vi "Strafe Correction.vi"() -> ()   [LabVIEW 2018]
uses:
  Global Variables/Yaw.vi
  Global Variables/Strafe Correction TF.vi
  Global Variables/Follow Yaw.vi
  Global Variables/Strafe Correction Voltage.vi
  <vilib>/addons/control/pid/pid.llb/PID (DBL).vi
  <vilib>/addons/control/pid/NI_PID_pid.lvlib
panel:
  in  "error in (no error)":errorcluster
  in  "PID gains":T1={"proportional gain (Kc)"=1.0, "integral time (Ti, min)"=0.01, "derivative time (Td, min)"=0.0} {"derivative time (Td, min)" format="%.3f"; "integral time (Ti, min)" format="%.3f"; "proportional gain (Kc)" format="%.3f"}
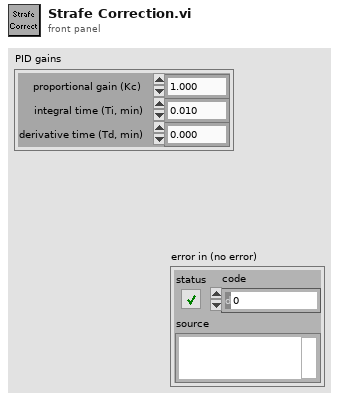
[diagram p1: front panel]
types:
  T1 = cluster{"proportional gain (Kc)":dbl, "integral time (Ti, min)":dbl, "derivative time (Td, min)":dbl}
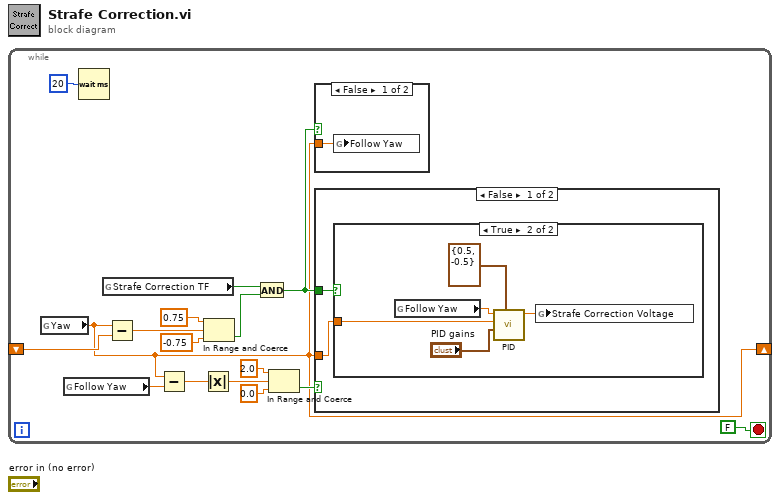
[diagram p0: block diagram]
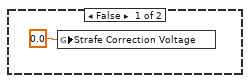
[diagram p3: hidden frame]
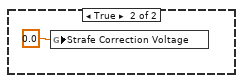
[diagram p4: hidden frame]
diagram:
  n1 = while {
    shift-right: [w1] -> _
    shift-left: _ -> [w8]
    stop <- FALSE stop-if-true
    n2 = global read "Yaw.vi" "Yaw"() -> (w1:dbl)
    n3 = global read "Follow Yaw.vi" "Follow Yaw"() -> (w14:dbl)
    n4 = Wait (ms)(milliseconds to wait=u32 20) -> ()  [unwired: 1 out]
    n5 = global read "Strafe Correction TF.vi" "Strafe Correction TF"() -> (w13:bool)
    n6 = Subtract(x=w1, y=w8) -> (x-y=w7:dbl)
    n7 = Subtract(x=w1, y=w14) -> (x-y=w10:dbl)
    n8 = Absolute Value(x=w10) -> (abs(x)=w9:dbl)
    n9 = In Range and Coerce(upper limit=0.75, x=w7, lower limit=-0.75) -> (In Range?=w3:bool)  [unwired: 1 out]
    n10 = And(x=w13, y=w3) -> (x .and. y?=w2:bool)
    n11 = In Range and Coerce(upper limit=2.0, x=w9, lower limit=0.0) -> (In Range?=w4:bool)  [unwired: 1 out]
    n12 = case shown="False" w2 {
      tunnel: w1 -> [w17 _]
      frame False {
        n13 = global write "Follow Yaw.vi" "Follow Yaw"(w17) -> ()
      }
      frame True {
      }
    }
    n14 = case shown="False" w4 {
      tunnel: w2 -> [w19 _]
      tunnel: w1 -> [w18 _]
      frame False {
        n15 = case shown="True" w19 {
          tunnel: w18 -> [_ w21]
          frame False {
            n16 = global write "Strafe Correction Voltage.vi" "Strafe Correction Voltage"(0.0 ("Strafe Correction Voltage")) -> ()
          }
          frame True {
            n17 = global read "Follow Yaw.vi" "Follow Yaw"() -> (w23:dbl)
            n18 = call-poly <vilib>:"PID.vi"("output range"=cluster{"output high":dbl, "output low":dbl} {"output high"=0.5, "output low"=-0.5}, "PID gains"="PID gains", "process variable"=w21, "setpoint"=w23) -> ("output"=w24:dbl)  [unwired: 6 in, 1 out]
            n19 = global write "Strafe Correction Voltage.vi" "Strafe Correction Voltage"(w24) -> ()
          }
        }
      }
      frame True {
        n20 = global write "Strafe Correction Voltage.vi" "Strafe Correction Voltage"(0.0 ("Strafe Correction Voltage")) -> ()
      }
    }
  }
